vi "Lab5_LV_TempSensor.vi"() -> (2 "Temperature Slider Value":dbl)   [LabVIEW 2014]
panel:
  in  "Temperature Slider":dbl(slide)=10.0 scale=0.0..125.0
  # "Simulate (Pretend) Reading Temperature from a Sensor"
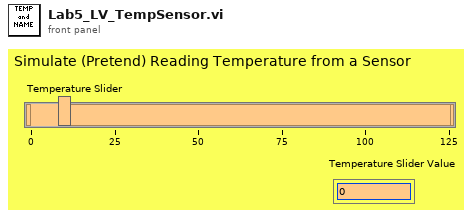
[diagram p1: front panel]
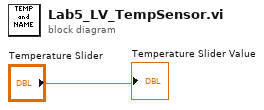
[diagram p0: block diagram]
diagram:
  "Temperature Slider Value" <- "Temperature Slider"
